vi "New Quiz.vi"(5 "Prob Ref":refnum<vi>[](array[refnum]), 7 "Quiz Data":T3[](array[typedef])=[{"Question Type"=enum."Text", "Solution Type"=enum."Number", "Question"={"Text"="", "Image"=bytes[0]}, "Solution"={"Numeric"={"Min"=0.0, "Max"=0.0, "Sig Figs"=0, "Sig Figs?"=FALSE}, "Text"="", "True/False"=FALSE, "MultiSelect"={"A"=TRUE, "B"=FALSE, "C"=FALSE, "D"=FALSE, "E"=FALSE}, "MultiText"=[], "Text Case Match"=FALSE}, "Stored Solution"={"Numeric"=0.0, "Text"="", "Multi"={"A"=TRUE, "B"=FALSE, "C"=FALSE, "D"=FALSE, "E"=FALSE}, "Radio"=enum."A", "True/False"=enum."True", "Short Answer"=""}, "Button Color"=0}, {"Question Type"=enum."Text", "Solution Type"=enum."Number", "Question"={"Text"="", "Image"=bytes[0]}, "Solution"={"Numeric"={"Min"=0.0, "Max"=0.0, "Sig Figs"=0, "Sig Figs?"=FALSE}, "Text"="", "True/False"=FALSE, "MultiSelect"={"A"=TRUE, "B"=FALSE, "C"=FALSE, "D"=FALSE, "E"=FALSE}, "MultiText"=[], "Text Case Match"=FALSE}, "Stored Solution"={"Numeric"=0.0, "Text"="", "Multi"={"A"=TRUE, "B"=FALSE, "C"=FALSE, "D"=FALSE, "E"=FALSE}, "Radio"=enum."A", "True/False"=enum."True", "Short Answer"=""}, "Button Color"=0}, {"Question Type"=enum."Text", "Solution Type"=enum."Number", "Question"={"Text"="", "Image"=bytes[0]}, "Solution"={"Numeric"={"Min"=0.0, "Max"=0.0, "Sig Figs"=0, "Sig Figs?"=FALSE}, "Text"="", "True/False"=FALSE, "MultiSelect"={"A"=TRUE, "B"=FALSE, "C"=FALSE, "D"=FALSE, "E"=FALSE}, "MultiText"=[], "Text Case Match"=FALSE}, "Stored Solution"={"Numeric"=0.0, "Text"="", "Multi"={"A"=TRUE, "B"=FALSE, "C"=FALSE, "D"=FALSE, "E"=FALSE}, "Radio"=enum."A", "True/False"=enum."True", "Short Answer"=""}, "Button Color"=0}, {"Question Type"=enum."Text", "Solution Type"=enum."Number", "Question"={"Text"="", "Image"=bytes[0]}, "Solution"={"Numeric"={"Min"=0.0, "Max"=0.0, "Sig Figs"=0, "Sig Figs?"=FALSE}, "Text"="", "True/False"=FALSE, "MultiSelect"={"A"=TRUE, "B"=FALSE, "C"=FALSE, "D"=FALSE, "E"=FALSE}, "MultiText"=[], "Text Case Match"=FALSE}, "Stored Solution"={"Numeric"=0.0, "Text"="", "Multi"={"A"=TRUE, "B"=FALSE, "C"=FALSE, "D"=FALSE, "E"=FALSE}, "Radio"=enum."A", "True/False"=enum."True", "Short Answer"=""}, "Button Color"=0}, {"Question Type"=enum."Text", "Solution Type"=enum."Number", "Question"={"Text"="", "Image"=bytes[0]}, "Solution"={"Numeric"={"Min"=0.0, "Max"=0.0, "Sig Figs"=0, "Sig Figs?"=FALSE}, "Text"="", "True/False"=FALSE, "MultiSelect"={"A"=TRUE, "B"=FALSE, "C"=FALSE, "D"=FALSE, "E"=FALSE}, "MultiText"=[], "Text Case Match"=FALSE}, "Stored Solution"={"Numeric"=0.0, "Text"="", "Multi"={"A"=TRUE, "B"=FALSE, "C"=FALSE, "D"=FALSE, "E"=FALSE}, "Radio"=enum."A", "True/False"=enum."True", "Short Answer"=""}, "Button Color"=0}], 8 "Error In":errorcluster, 9 "Quiz Solution":T1={"Numeric"=0.0, "Text"="", "Multi"={"A"=TRUE, "B"=FALSE, "C"=FALSE, "D"=FALSE, "E"=FALSE}, "Radio"=enum."A", "True/False"=enum."True", "Short Answer"=""}, 10 "Index":i32, 11 "Mode":T2) -> (0 "Error Out":errorcluster, 2 "Grade String":string)   [LabVIEW 2012]
uses:
  Controls/Quiz Info.ctl
  Controls/Quiz Solution.ctl
  Controls/Quiz Mode.ctl
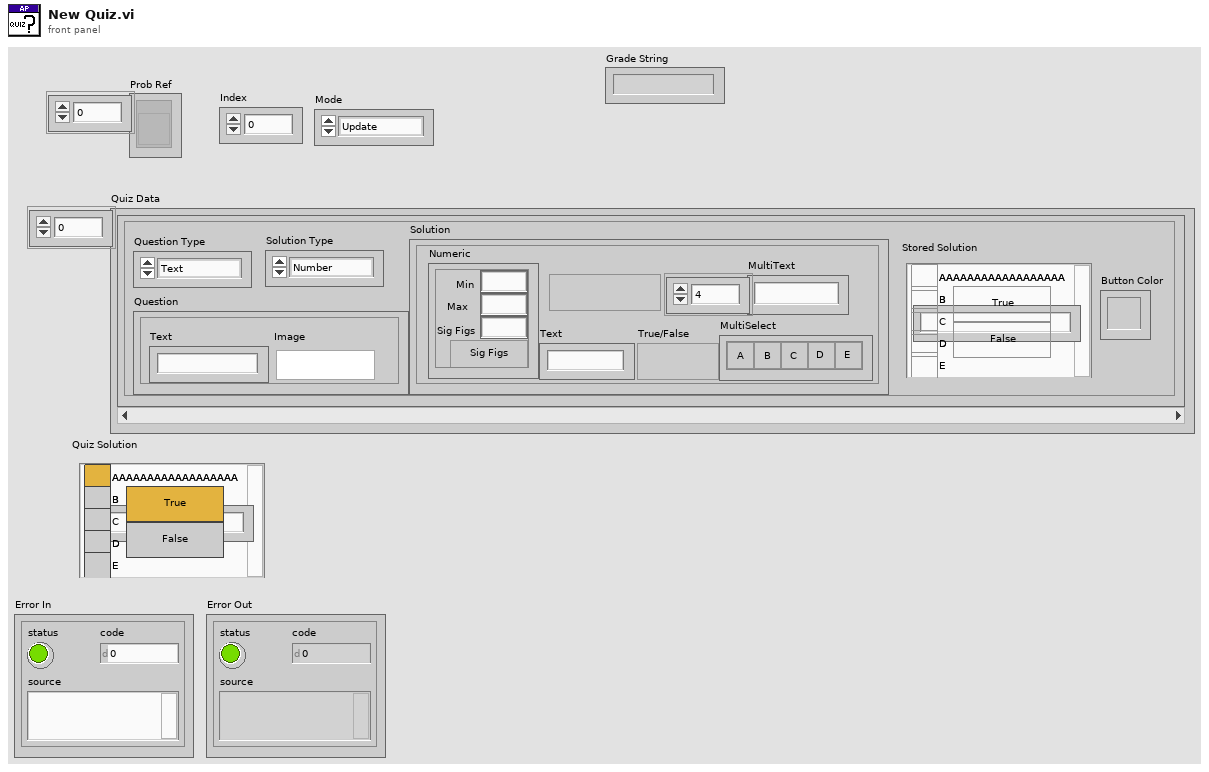
[diagram p1: front panel]
types:
  T1 = typedef "Quiz Solution.ctl" = cluster{"Numeric":dbl, "Text":string, "Multi":cluster{"A":bool, "B":bool, "C":bool, "D":bool, "E":bool}, "Radio":enum32{"No Selection", "A", "B", "C", "D", "E"}, "True/False":enum32{"No Selection", "True", "False"}, "Short Answer":string}
  T2 = typedef "Quiz Mode.ctl" = enum16{"Update", "Store Solution", "Grade"}
  T3 = typedef "Quiz Info.ctl" = cluster{"Question Type":enum16{"Text", "Image", "Text&Image"}, "Solution Type":enum16{"Number", "Text", "MultiChoice", "Radio", "T/F", "Paragraph"}, "Question":cluster{"Text":string, "Image":picture}, "Solution":cluster{"Numeric":cluster{"Min":dbl, "Max":dbl, "Sig Figs":i32, "Sig Figs?":bool}, "Text":string, "True/False":bool, "MultiSelect":cluster{"A":bool, "B":bool, "C":bool, "D":bool, "E":bool}, "MultiText":string[], "Text Case Match":bool}, "Stored Solution":T1, "Button Color":u32}
  T4 = enum8{"Enabled", "Disabled", "Disabled and Grayed Out"}
  T5 = enum16{"Number", "Text", "MultiChoice", "Radio", "T/F", "Paragraph"}
  T6 = cluster{"Numeric":cluster{"Min":dbl, "Max":dbl, "Sig Figs":i32, "Sig Figs?":bool}, "Text":string, "True/False":bool, "MultiSelect":cluster{"A":bool, "B":bool, "C":bool, "D":bool, "E":bool}, "MultiText":string[], "Text Case Match":bool}
  T7 = cluster{"A":bool, "B":bool, "C":bool, "D":bool, "E":bool}
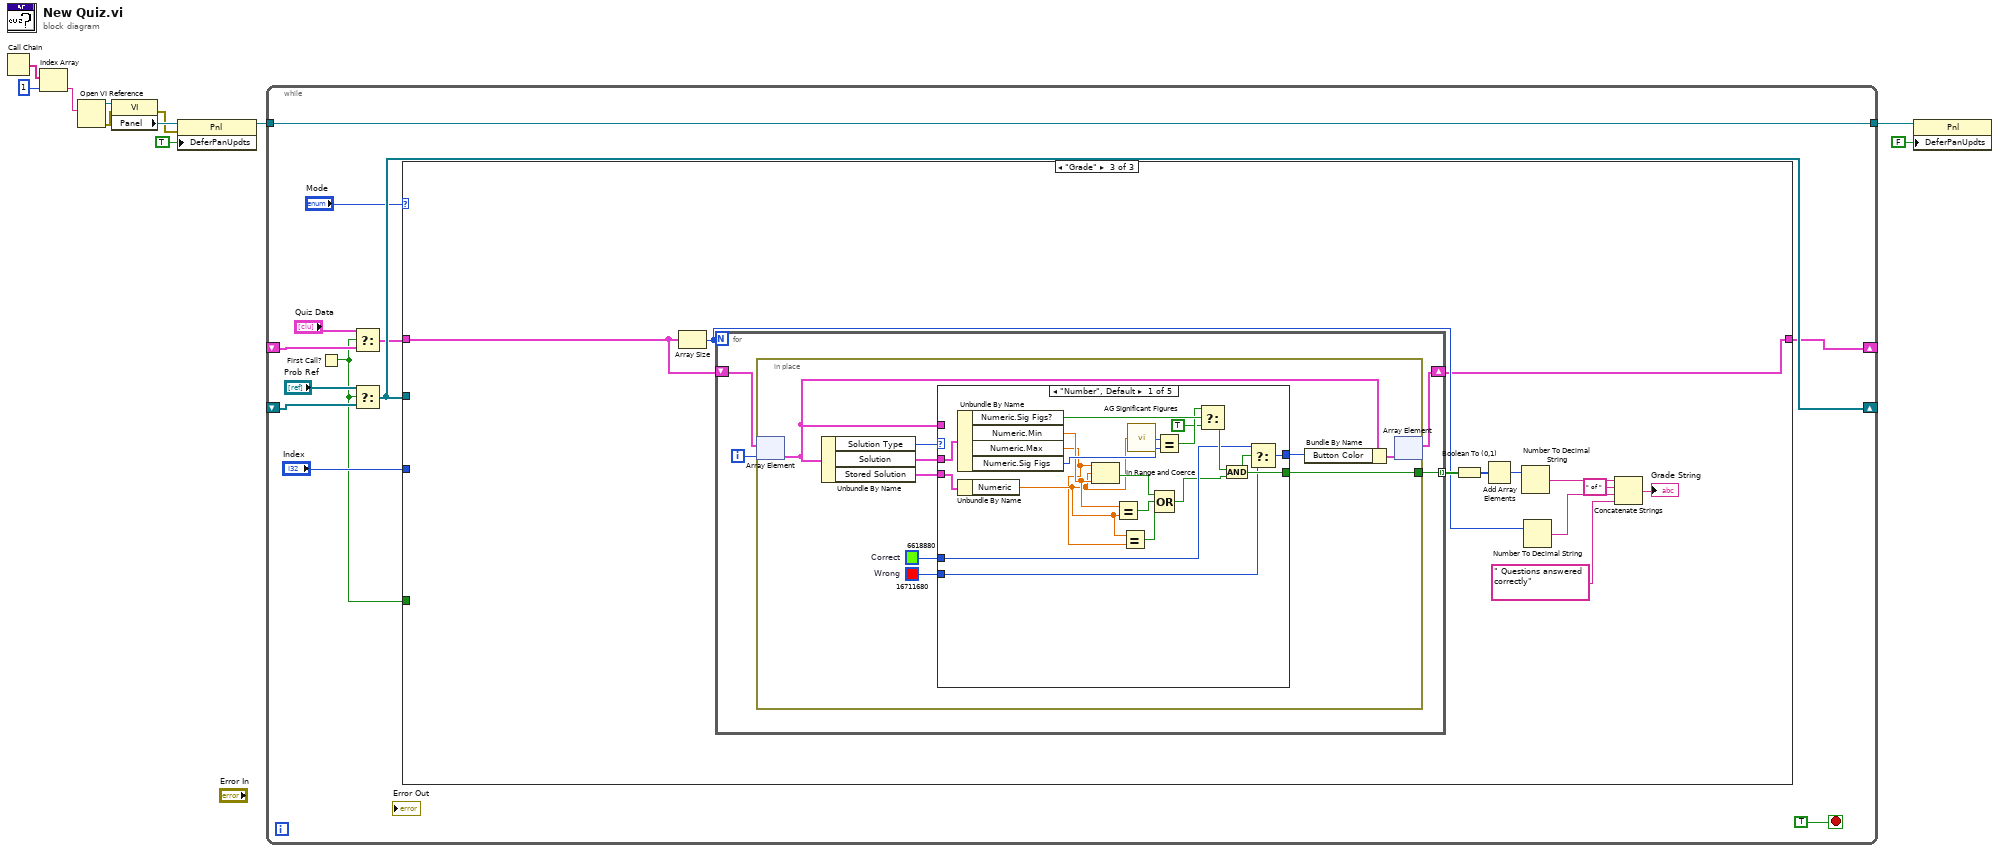
[diagram p0: block diagram]
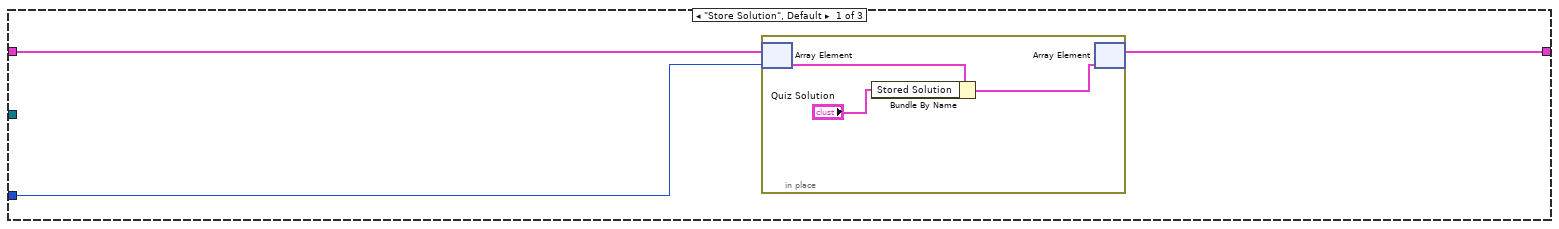
[diagram p2: hidden frame]
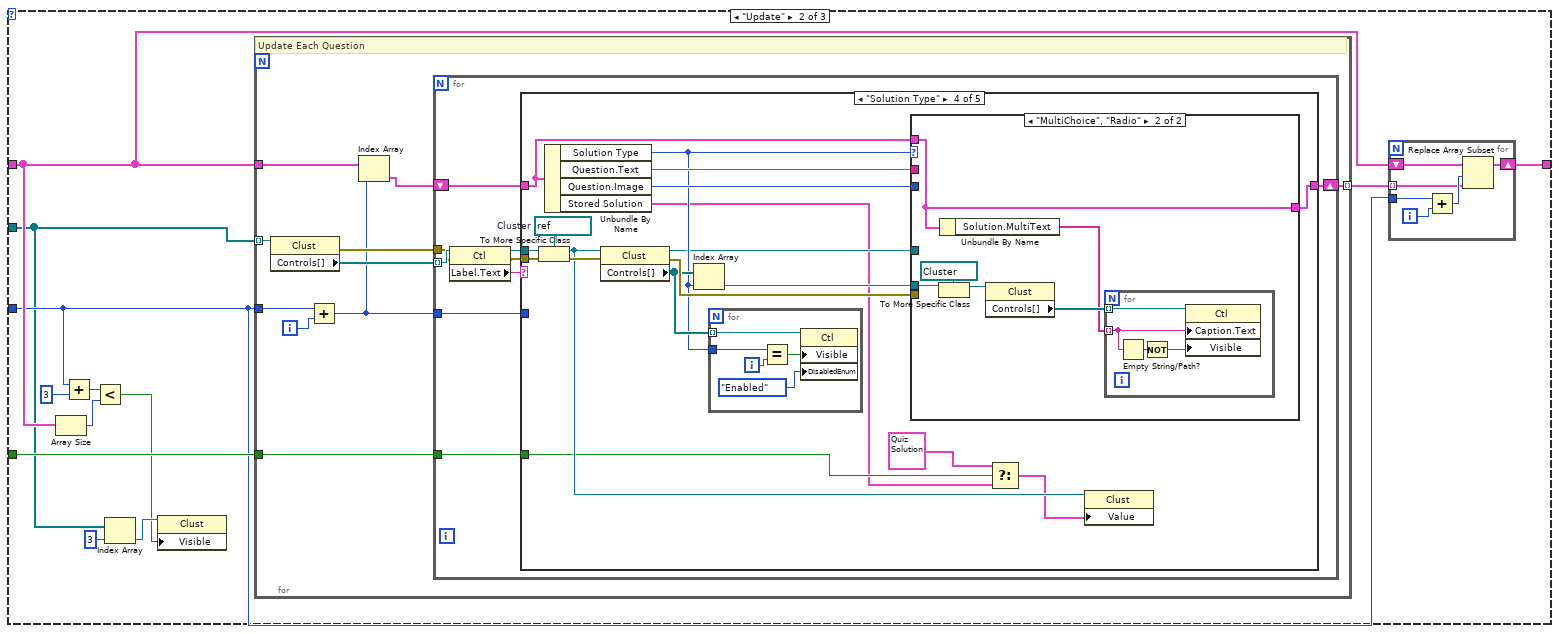
[diagram p3: hidden frame]
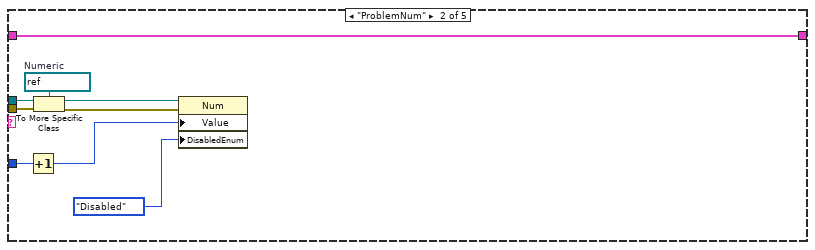
[diagram p5: hidden frame]
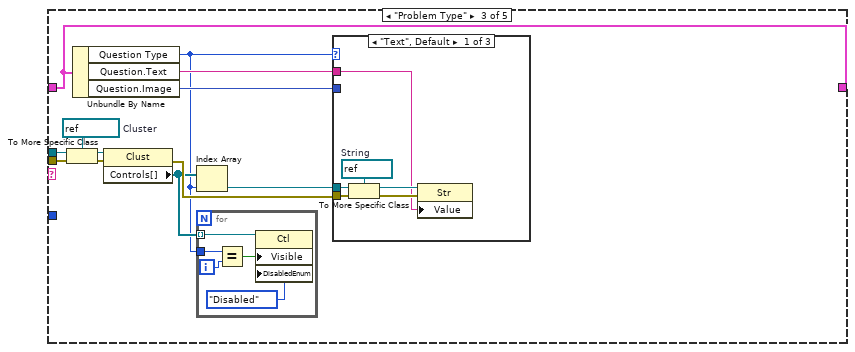
[diagram p6: hidden frame]
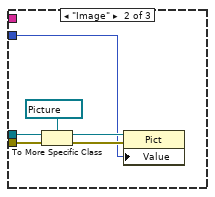
[diagram p7: hidden frame]
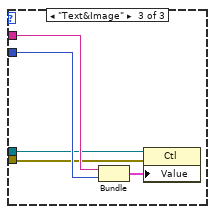
[diagram p8: hidden frame]
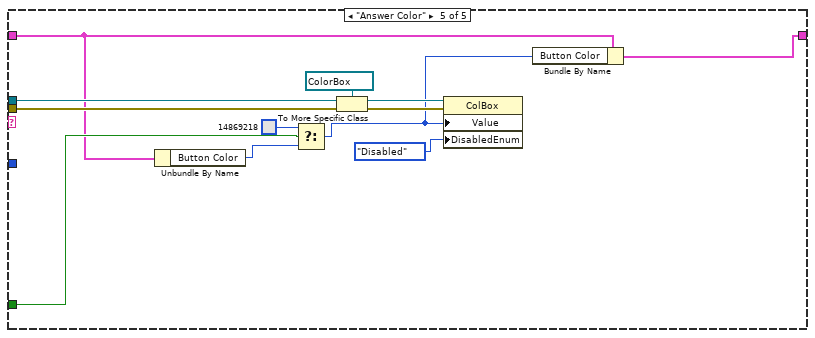
[diagram p10: hidden frame]
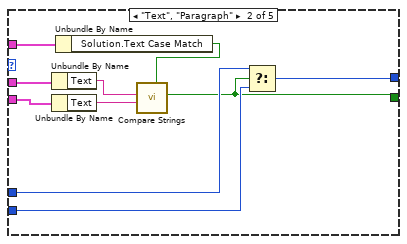
[diagram p11: hidden frame]
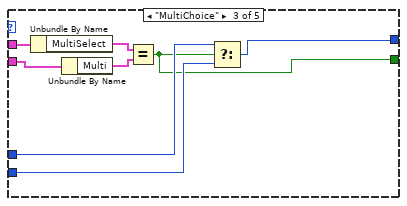
[diagram p12: hidden frame]
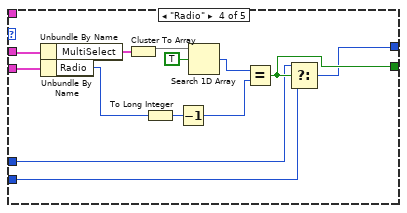
[diagram p13: hidden frame]
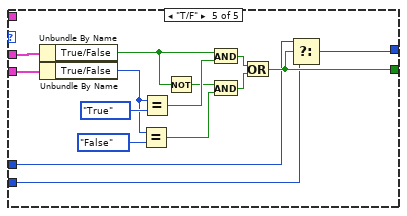
[diagram p14: hidden frame]
diagram:
  n1 = Call Chain() -> (call chain=w6:string[])
  n2 = Index Array(array=w6, index=1) -> (element=w4:string)
  n3 = Open VI Reference(vi path=w4) -> (vi reference=w9:refnum<vi>, error out=w7:errorcluster)  [unwired: 5 in]
  n4 = property class="VI"(reference=w9, error in=w7) -> (error out=w8:errorcluster, "Panel"=w11:refnum<vi>)  [unwired: 1 out]
  n5 = property class="Pnl"(reference=w11, error in=w8, "DeferPanUpdts"=TRUE ("Defer Panel Updates")) -> (reference out=w2:refnum<vi>)  [unwired: 1 out]
  n6 = while {
    shift-right: [w17] -> _
    shift-left: _ -> [w22]
    shift-right: [w19] -> _
    shift-left: _ -> [w20]
    tunnel: w2 -> [w12]
    tunnel: [w12] -> w1
    stop <- TRUE stop-if-true
    n7 = First Call?() -> (First Call?: T/F=w14:bool)
    n8 = Select(t="Quiz Data", s=w14, f=w22) -> (s? t:f=w18:T3[])
    n9 = Select(t="Prob Ref", s=w14, f=w20) -> (s? t:f=w19:refnum<vi>[])
    n10 = case shown="\"Grade\"" "Mode" {
      tunnel: w19 -> [_ w33 _]
      tunnel: w18 -> [w26 w36 w167]
      tunnel: [w24 w41 w157] -> w17
      tunnel: "Index" -> [w25 w35 _]
      tunnel: w14 -> [_ w39 _]
      frame "Store Solution", Default {
        n11 = in-place {
          n12 = in-place-array #1(w26, w25) -> (w29:T3)
          n13 = Bundle By Name(cluster=w29, "Stored Solution"="Quiz Solution") -> (w27:T3)
          n14 = in-place-array #1(w27) -> (w24:T3[])  [unwired: 1 out]
        }
      }
      frame "Update" {
        n15 = Array Size(array=w36) -> (size(s)=w38:i32)
        n16 = Add(x=w35, y=3) -> (x+y=w37:i32)
        n17 = Less?(x=w37, y=w38) -> (x < y?=w30:bool)
        n18 = Index Array(array=w33, index=3) -> (element=w31:refnum<vi>)
        n19 = property class="Clust"(reference=w31, "Visible"=w30) -> ()  [unwired: 1 in, 2 out]
        n20 = for {
          tunnel: w33 -> [w57] mode=indexing
          tunnel: w35 -> [w48]
          tunnel: [w53] -> w40 mode=indexing
          tunnel: w36 -> [w49]
          tunnel: w39 -> [w50]
          i -> [w54]
          # "Update Each Question"
          n21 = property class="Clust"(reference=w57) -> (error out=w55:errorcluster, "Controls[]"=w56:refnum<vi>[])  [unwired: 1 in, 1 out]
          n22 = Add(x=w48, y=w54) -> (x+y=w52:i32)
          n23 = Index Array(array=w49, index=w52) -> (element=w51:T3)
          n24 = for {
            tunnel: w56 -> [w66] mode=indexing
            tunnel: w52 -> [w61]
            tunnel: w55 -> [w62]
            shift-right: [w59] -> w53
            shift-left: w51 -> [w60]
            tunnel: w50 -> [w58]
            n25 = property class="Ctl"(reference=w66, error in=w62) -> (reference out=w64:refnum<vi>, error out=w63:errorcluster, "Label.Text"=w65:string)
            n26 = case shown="\"Solution Type\"" w65 {
              tunnel: w64 -> [_ w75 w85 w125 w156]
              tunnel: w63 -> [_ w72 w86 w126 w155]
              tunnel: w61 -> [_ w71 _ _ _]
              tunnel: w60 -> [w67 w69 w77 w118 w147]
              tunnel: [w67 w69 w77 w117 w146] -> w59
              tunnel: w58 -> [_ _ _ w114 w150]
              frame "NULL", Default {
              }
              frame "ProblemNum" {
                w74 = refnum<vi> refnum  # Numeric
                n27 = Increment(x=w71) -> (x+1=w70:i32)
                n28 = To More Specific Class(target class=w74, reference=w75, error in=w72) -> (specific class reference=w76:refnum<vi>, error out=w73:errorcluster)
                n29 = property class="Num"(reference=w76, error in=w73, "Value"=w70, "DisabledEnum"=T4."Disabled" ("Disabled")) -> ()  [unwired: 2 out]
              }
              frame "Problem Type" {
                w84 = refnum<vi> refnum  # Cluster
                n30 = To More Specific Class(target class=w84, reference=w85, error in=w86) -> (specific class reference=w83:refnum<vi>, error out=w82:errorcluster)
                n31 = Unbundle By Name(w77) -> ("Question Type"=w78:enum16{"Text", "Image", "Text&Image"}, "Question.Text"=w88:string, "Question.Image"=w87:picture)
                n32 = property class="Clust"(reference=w83, error in=w82) -> (error out=w80:errorcluster, "Controls[]"=w79:refnum<vi>[])  [unwired: 1 out]
                n33 = Index Array(array=w79, index=w78) -> (element=w81:refnum<vi>)
                n34 = for {
                  tunnel: w79 -> [w93] mode=indexing
                  tunnel: w78 -> [w91]
                  i -> [w92]
                  n35 = Equal?(x=w91, y=w92) -> (x = y?=w90:bool)
                  n36 = property class="Ctl"(reference=w93, "Visible"=w90, "DisabledEnum"=T4."Disabled" ("Disabled")) -> ()  [unwired: 1 in, 2 out]
                }
                n37 = case shown="\"Text\", Default" w78 {
                  tunnel: w88 -> [w94 _ w110]
                  tunnel: w87 -> [_ w100 w109]
                  tunnel: w81 -> [w99 w105 w107]
                  tunnel: w80 -> [w97 w104 w106]
                  frame "Text", Default {
                    w98 = refnum<vi> refnum  # String
                    n38 = To More Specific Class(target class=w98, reference=w99, error in=w97) -> (specific class reference=w96:refnum<vi>, error out=w95:errorcluster)
                    n39 = property class="Str"(reference=w96, error in=w95, "Value"=w94) -> ()  [unwired: 2 out]
                  }
                  frame "Image" {
                    n40 = To More Specific Class(target class=refnum<vi> refnum ("Image"), reference=w105, error in=w104) -> (specific class reference=w102:refnum<vi>, error out=w101:errorcluster)
                    n41 = property class="Pict"(reference=w102, error in=w101, "Value"=w100) -> ()  [unwired: 2 out]
                  }
                  frame "Text&Image" {
                    n42 = Bundle("Text"=w110, "Image"=w109) -> (w108:cluster{"Text":string, "Image":picture})  [unwired: 1 in]
                    n43 = property class="Ctl"(reference=w107, error in=w106, "Value"=w108) -> ()  [unwired: 2 out]
                  }
                }
              }
              frame "Solution Type" {
                w124 = refnum<vi> refnum  # Cluster
                n44 = To More Specific Class(target class=w124, reference=w125, error in=w126) -> (specific class reference=w115:refnum<vi>, error out=w123:errorcluster)
                n45 = Unbundle By Name(w118) -> ("Solution Type"=w119:T5, "Question.Text"=w128:string, "Question.Image"=w127:picture, "Stored Solution"=w111:T1)
                n46 = property class="Clust"(reference=w115, error in=w123) -> (reference out=w116:refnum<vi>, error out=w121:errorcluster, "Controls[]"=w120:refnum<vi>[])
                n47 = Index Array(array=w120, index=w119) -> (element=w122:refnum<vi>)
                n48 = for {
                  tunnel: w120 -> [w133] mode=indexing
                  tunnel: w119 -> [w131]
                  i -> [w132]
                  n49 = Equal?(x=w131, y=w132) -> (x = y?=w129:bool)
                  n50 = property class="Ctl"(reference=w133, "Visible"=w129, "DisabledEnum"=T4."Enabled" ("Disabled")) -> ()  [unwired: 1 in, 2 out]
                }
                n51 = case shown="\"MultiChoice\", \"Radio\"" w119 {
                  tunnel: w128 -> [_ _]
                  tunnel: w127 -> [_ _]
                  tunnel: w122 -> [_ w140]
                  tunnel: w121 -> [_ _]
                  tunnel: w118 -> [w134 w135]
                  tunnel: [w134 w135] -> w117
                  tunnel: w116 -> [_ _]
                  frame "T/F", Default {
                  }
                  frame "MultiChoice", "Radio" {
                    n52 = To More Specific Class(target class=refnum<vi> refnum ("True/False"), reference=w140) -> (specific class reference=w139:refnum<vi>)  [unwired: 1 in, 1 out]
                    n53 = Unbundle By Name(w135) -> ("Solution.MultiText"=w136:string[])
                    n54 = property class="Clust"(reference=w139) -> ("Controls[]"=w137:refnum<vi>[])  [unwired: 1 in, 2 out]
                    n55 = for {
                      tunnel: w137 -> [w144] mode=indexing
                      tunnel: w136 -> [w143] mode=indexing
                      n56 = Empty String/Path?(string/path=w143) -> (empty?=w141:bool)
                      n57 = Not(x=w141) -> (.not. x?=w142:bool)
                      n58 = property class="Ctl"(reference=w144, "Caption.Text"=w143, "Visible"=w142) -> ()  [unwired: 1 in, 2 out]
                    }
                  }
                }
                n59 = Select(t=T1 {"Numeric"=0.0, "Text"="", "Multi"={"A"=FALSE, "B"=FALSE, "C"=FALSE, "D"=FALSE, "E"=FALSE}, "Radio"=enum."No Selection", "True/False"=enum."No Selection", "Short Answer"=""} ("Solution Type"), s=w114, f=w111) -> (s? t:f=w112:T1)
                n60 = property class="Clust"(reference=w115, "Value"=w112) -> ()  [unwired: 1 in, 2 out]
              }
              frame "Answer Color" {
                n61 = Unbundle By Name(w147) -> ("Button Color"=w148:u32)
                n62 = Select(t=u32 14869218, s=w150, f=w148) -> (s? t:f=w145:u32)
                n63 = To More Specific Class(target class=refnum<vi> refnum ("Answer Color"), reference=w156, error in=w155) -> (specific class reference=w153:refnum<vi>, error out=w152:errorcluster)
                n64 = property class="ColBox"(reference=w153, error in=w152, "Value"=w145, "DisabledEnum"=T4."Disabled" ("Disabled")) -> ()  [unwired: 2 out]
                n65 = Bundle By Name(cluster=w147, "Button Color"=w145) -> (w146:T3)
              }
            }
          }
        }
        n66 = for {
          shift-right: [w46] -> w41
          shift-left: w36 -> [w47]
          tunnel: w35 -> [w45]
          tunnel: w40 -> [w42] mode=indexing
          i -> [w44]
          n67 = Add(x=w45, y=w44) -> (x+y=w43:i32)
          n68 = Replace Array Subset(array=w47, new element=w42, index=w43) -> (w46:T3[])
        }
      }
      frame "Grade" {
        n69 = Array Size(array=w167) -> (size(s)=w163:i32)
        n70 = for {
          N: w163 -> [_]
          tunnel: [w171] -> w165 mode=indexing
          shift-right: [w168] -> w157
          shift-left: w167 -> [w170]
          i -> [w169]
          n71 = in-place {
            in-place-border: [w177] -> w171
            w172 = u32 6618880  # Correct
            w173 = u32 16711680  # Wrong
            n72 = in-place-array #2(w170, w169) -> (w175:T3)
            n73 = Unbundle By Name(w175) -> ("Solution Type"=w180:T5, "Solution"=w179:T6, "Stored Solution"=w178:T1)
            n74 = case shown="\"Number\", Default" w180 {
              tunnel: w179 -> [w198 w209 w217 w229 w245]
              tunnel: w178 -> [w199 w208 w216 w230 w244]
              tunnel: w175 -> [_ w207 _ _ _]
              tunnel: [w190 w200 w210 w224 w235] -> w177
              tunnel: [w191 w206 w211 w221 w232] -> w174
              tunnel: w173 -> [w189 w205 w212 w222 w233]
              tunnel: w172 -> [w188 w204 w213 w223 w234]
              frame "Number", Default {
                n75 = Unbundle By Name(w198) -> ("Numeric.Sig Figs?"=w195:bool, "Numeric.Min"=w187:dbl, "Numeric.Max"=w181:dbl, "Numeric.Sig Figs"=w196:i32)
                n76 = Unbundle By Name(w199) -> ("Numeric"=w182:dbl)
                n77 = In Range and Coerce(upper limit=w181, x=w182, lower limit=w187) -> (In Range?=w184:bool)  [unwired: 1 out]
                n78 = Equal?(x=w187, y=w182) -> (x = y?=w186:bool)
                n79 = Equal?(x=w182, y=w181) -> (x = y?=w185:bool)
                n80 = call "AG Significant Figures.vi"("Number"=w182) -> ("Sig Figs"=w197:i32)
                n81 = Compound Arithmetic op=OR(w184, w186, w185) -> (w183:bool)
                n82 = Equal?(x=w197, y=w196) -> (x = y?=w194:bool)
                n83 = Select(t=w194, s=w195, f=TRUE) -> (s? t:f=w192:bool)
                n84 = And(x=w192, y=w183) -> (x .and. y?=w190:bool)
                n85 = Select(t=w188, s=w190, f=w189) -> (s? t:f=w191:u32)
              }
              frame "Text", "Paragraph" {
                n86 = Unbundle By Name(w209) -> ("Text"=w203:string)
                n87 = Unbundle By Name(w208) -> ("Text"=w202:string)
                n88 = Unbundle By Name(w207) -> ("Solution.Text Case Match"=w201:bool)
                n89 = call "Compare Strings.vi"("ignore case? (T)"=w201, "String2"=w202, "String1"=w203) -> ("Match"=w200:bool)  [unwired: 8 in]
                n90 = Select(t=w204, s=w200, f=w205) -> (s? t:f=w206:u32)
              }
              frame "MultiChoice" {
                n91 = Unbundle By Name(w217) -> ("MultiSelect"=w215:T7)
                n92 = Unbundle By Name(w216) -> ("Multi"=w214:T7)
                n93 = Equal?(x=w215, y=w214) -> (x = y?=w210:bool)
                n94 = Select(t=w213, s=w210, f=w212) -> (s? t:f=w211:u32)
              }
              frame "Radio" {
                n95 = Unbundle By Name(w229) -> ("MultiSelect"=w226:T7)
                n96 = Unbundle By Name(w230) -> ("Radio"=w219:enum32{"No Selection", "A", "B", "C", "D", "E"})
                n97 = Cluster To Array(cluster=w226) -> (array=w228:bool[])
                n98 = To Long Integer(number=w219) -> (32bit integer=w220:i32)
                n99 = Decrement(x=w220) -> (x-1=w218:i32)
                n100 = Search 1D Array(1D array=w228, element=TRUE) -> (index of element=w225:i32)  [unwired: 1 in]
                n101 = Equal?(x=w225, y=w218) -> (x = y?=w224:bool)
                n102 = Select(t=w223, s=w224, f=w222) -> (s? t:f=w221:u32)
              }
              frame "T/F" {
                n103 = Unbundle By Name(w245) -> ("True/False"=w237:bool)
                n104 = Unbundle By Name(w244) -> ("True/False"=w231:enum32{"No Selection", "True", "False"})
                n105 = Equal?(x=w231, y=enum32{"No Selection", "True", "False"}."False") -> (x = y?=w238:bool)
                n106 = Equal?(x=w231, y=enum32{"No Selection", "True", "False"}."True") -> (x = y?=w242:bool)
                n107 = Not(x=w237) -> (.not. x?=w236:bool)
                n108 = And(x=w237, y=w242) -> (x .and. y?=w241:bool)
                n109 = And(x=w236, y=w238) -> (x .and. y?=w239:bool)
                n110 = Or(x=w241, y=w239) -> (x .or. y?=w235:bool)
                n111 = Select(t=w234, s=w235, f=w233) -> (s? t:f=w232:u32)
              }
            }
            n112 = Bundle By Name(cluster=w175, "Button Color"=w174) -> (w176:T3)
            n113 = in-place-array #2(w176) -> (w168:T3[])  [unwired: 1 out]
          }
        }
        n114 = Boolean To (0,1)(Boolean=w165) -> (0, 1=w166:i16[])
        n115 = Add Array Elements(numeric array=w166) -> (sum=w164:i16)
        n116 = Number To Decimal String(number=w164) -> (decimal integer string=w162:string)  [unwired: 1 in]
        n117 = Number To Decimal String(number=w163) -> (decimal integer string=w160:string)  [unwired: 1 in]
        n118 = Concatenate Strings(w162, " of " ("string"), w160, " Questions answered correctly" ("string")) -> (→"Grade String":string)
      }
    }
  }
  n119 = property class="Pnl"(reference=w1, "DeferPanUpdts"=FALSE ("Defer Panel Updates")) -> ()  [unwired: 1 in, 2 out]
